vi "AlliGator Read IRFs & Fit Data HDF5 File Metadata.vi"(8 "error in (no error)":errorcluster, 11 "ref in":T1 format="%.0x") -> (0 "error out":errorcluster, 1 "File Metadata":string, 3 "ref out":T1 format="%.0x")   [LabVIEW 2021, in "AlliGator Decay Fit Parameter Map.lvlib"]
doc: "Reads Decay Fit Parameter Map metadata from HDF5 file."
uses:
  <vilib>/addons/h5labview2/base/hid_t.ctl
  <vilib>/addons/h5labview2/base/lib_path.vi
  <vilib>/addons/h5labview2/base/H5Equery.vi
  <vilib>/addons/h5labview2/dataset/H5Dread.llb/H5Dread.xnode
  AlliGator Decay Fit Parameter Map.lvlib
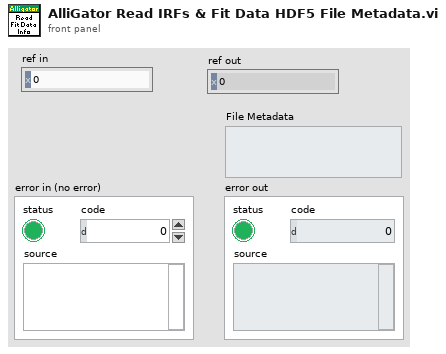
[diagram p1: front panel]
types:
  T1 = typedef "hid_t.ctl" = i64
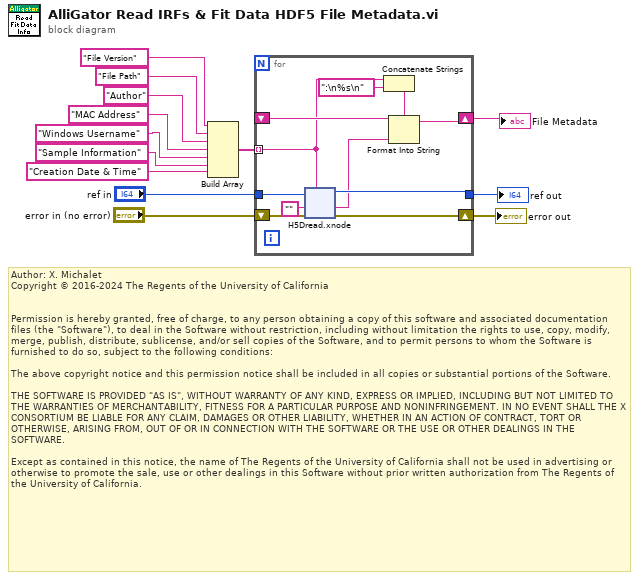
[diagram p0: block diagram]
diagram:
  # "Author: X. Michalet\nCopyright © 2016-2024 The Regents of the University of California\n \n\nPermission is hereby granted, free of charge, to any person obtaining a copy of this software and associated documentation files (the \"Software\"), to deal in the Software without restriction, including without limitation the rights to use, copy, modify, merge, publish, distribute, sublicense, and/or sell copies of the Software, and to permit persons to whom the Software is furnished to do so, subject to the following conditions:\n\nThe above copyright notice and this permission notice shall be included in all copies or substantial portions of the Software.\n\nTHE SOFTWARE IS PROVIDED \"AS IS\", WITHOUT WARRANTY OF ANY KIND, EXPRESS OR IMPLIED, INCLUDING BUT NOT LIMITED TO THE WARRANTIES OF MERCHANTABILITY, FITNESS FOR A PARTICULAR PURPOSE AND NONINFRINGEMENT. IN NO EVENT SHALL THE X CONSORTIUM BE LIABLE FOR ANY CLAIM, DAMAGES OR OTHER LIABILITY, WHETHER IN AN ACTION OF CONTRACT, TORT OR OTHERWISE, ARISING FROM, OUT OF OR IN CONNECTION WITH THE SOFTWARE OR THE USE OR OTHER DEALINGS IN THE SOFTWARE.\n\nExcept as contained in this notice, the name of The Regents of the University of California shall not be used in advertising or otherwise to promote the sale, use or other dealings in this Software without prior written authorization from The Regents of the University of California."
  n1 = Build Array("File Version" ("dataset name"), "File Path" ("dataset name"), "Author" ("dataset name"), "MAC Address" ("dataset name"), "Windows Username" ("dataset name"), "Sample Information" ("name"), "Creation Date & Time" ("dataset name")) -> (w6:string[])
  n2 = for {
    tunnel: w6 -> [w15] mode=indexing
    shift-right: [w22] -> w3
    shift-left: "error in (no error)" -> [w23]
    shift-right: [w17] -> w2
    shift-left: _ -> [w20]
    tunnel: "ref in" -> [w24]
    tunnel: [w21] -> w4
    n3 = xnode "H5Dread.xnode"("dataset name (this)"=w15, "error in (no error)"=w23, "default"="", "ref in"=w24) -> ("error out"=w22:errorcluster, "data"=w16:string, "ref out"=w21:T1)  [unwired: 2 in, 1 out]
    n4 = Concatenate Strings(w15, ":\n%s\n" ("string")) -> (w18:string)
    n5 = Format Into String(format string=w18, initial string=w20, w16) -> (resulting string=w17:string)  [unwired: 1 in, 1 out]
  }
  "error out" <- w3
  "ref out" <- w4
  "File Metadata" <- w2
